vi "VI Properties Editor.vi"() -> ()   [LabVIEW 2023, in "VI Properties Editor.lvlib"]
doc: "Displays a window to add and edit properties of VIs in a streamlined way."
uses:
  VI Properties Editor.lvlib
  CTLs/VI Properties Editor State Data.ctl
  CTLs/VI Data.ctl
  CTLs/VI Properties.ctl
  <vilib>/picture/picture.llb/imagedata.ctl
  CTLs/Control Properties.ctl
  CTLs/VI Properties Editor Front Panel Controls.ctl
  CTLs/Config.ctl
  <vilib>/Utility/miscctls.llb/LVSelectionTypeDef.ctl
  <vilib>/ErrorRing/Error Ring.xnode
  SubVIs/FaKI SM.lvlib
panel:
  in  "Same Title as VI?":bool caption="Same as VI name"
  in  "Window Title":string
  in  "Add Copyright":bool
  out "Inline?":bool
  out "Reentrant?":bool
  in  "Prompt?":bool
  in  "Set all VIs":bool
  in  "error in (no error)":errorcluster
  in  "Controls":string[][](table)
  in  "Indicators":string[][](table)
  in  "Help Tag":string
  in  "Help Path":string
  out "Path to VI":string
  in  "VI Description":string
  out "VI Conn Pane":picture
  in  "Listbox with VIs":i32(listbox)=-1 caption="Select a VI to View/Edit Properties:"
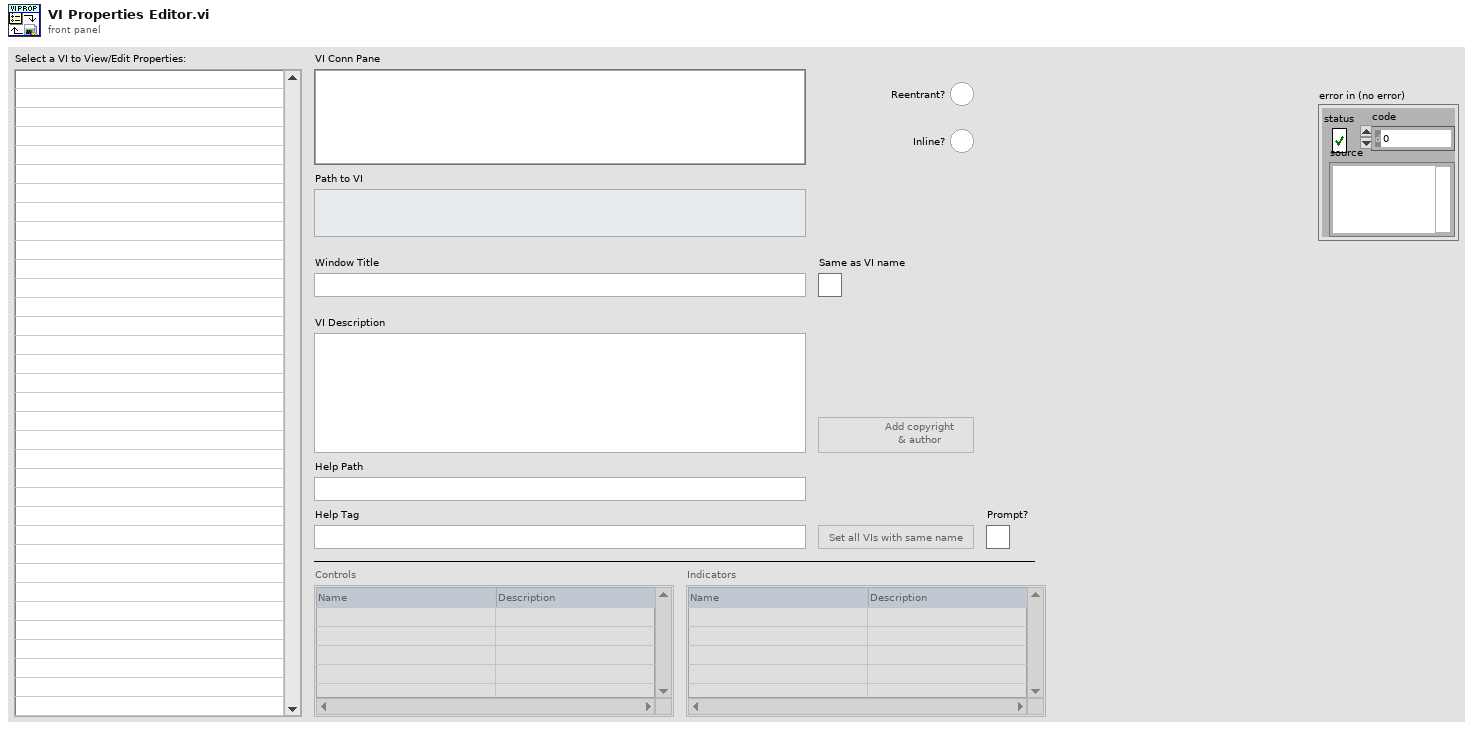
[diagram p1: front panel]
types:
  T1 = typedef "VI Properties Editor.lvlib/VI Properties Editor State Data.ctl" = cluster{"Core":cluster{"Current VI Reference":refnum<vi>, "Close Panel on Exit?":bool}, "New VI Data":T2[], "Saved VI Data":T2[], "Current Folder":path, "FP":T6, "Config Path":path, "Config":T7, "Desc Selection":T8}
  T2 = typedef "VI Properties Editor.lvlib/VI Data.ctl" = cluster{"VI":T3, "Ctl Properties":T5[]}
  T3 = typedef "VI Properties Editor.lvlib/VI Properties.ctl" = cluster{"Name":string, "Path":path, "Type":enum32{"invalid VI type", "Standard VI", "Control VI", "Global VI", "Polymorphic VI", "Configuration VI", "SubSystem", "Facade VI", "Method VI", "Statechart Diagram VI"}, "Window Title":string, "Description":string, "Help Path":path, "Help Tag":string, "Custom Title?":bool, "Reentrant?":bool, "Inlined?":bool, "Conpane Img":T4}
  T4 = typedef "imagedata.ctl" = cluster{"image type":i32, "image depth":i32, "image":u8[], "mask":u8[], "colors":u32[], "Rectangle":cluster{"left":i16, "top":i16, "right":i16, "bottom":i16}}
  T5 = typedef "VI Properties Editor.lvlib/Control Properties.ctl" = cluster{"UID":i32, "Name":string, "Description":string, "Tip Strip":string, "Is Indicator?":bool}
  T6 = typedef "VI Properties Editor.lvlib/VI Properties Editor Front Panel Controls.ctl" = cluster{"VI Selected":i32, "Help Path":string, "Help Tag":string, "VI Desc":string, "Controls":string[][], "Indicators":string[][], "Window Title":string, "Same Title?":bool}
  T7 = typedef "VI Properties Editor.lvlib/Config.ctl" = cluster{"Copyright Path":path, "Abbreviate Names?":bool, "Format Bold Text?":bool}
  T8 = typedef "LVSelectionTypeDef.ctl" = cluster{"Selection Start":u32, "Selection End":u32}
  T9 = enum32{"Invalid", "Standard", "Closed", "Hidden", "Minimized", "Maximized"}
  T10 = enum32{"invalid app kind", "Development System", "Run Time System", "Student Edition", "Embedded LabVIEW", "Evaluation", "Custom"}
  T11 = enum32{"invalid VI type", "Standard VI", "Control VI", "Global VI", "Polymorphic VI", "Configuration VI", "SubSystem", "Facade VI", "Method VI", "Statechart Diagram VI"}
  T12 = enum8{"Enabled", "Disabled", "Disabled and Grayed Out"}
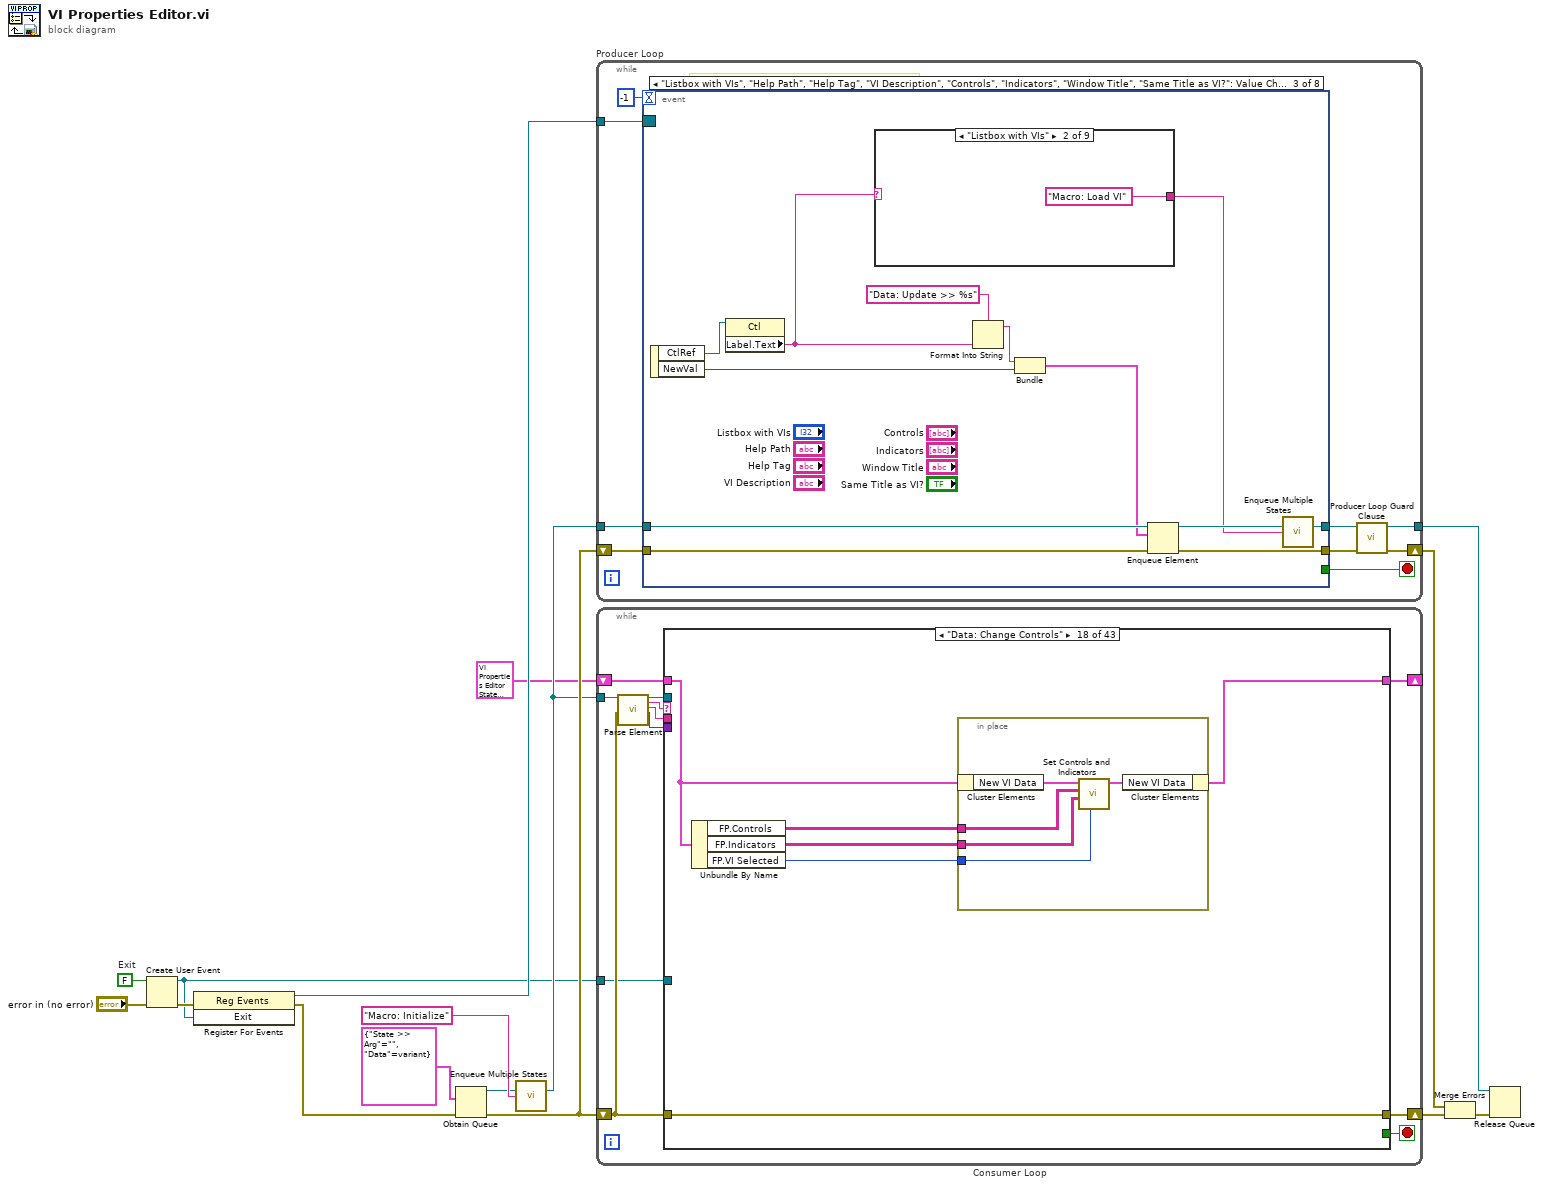
[diagram p0: block diagram]
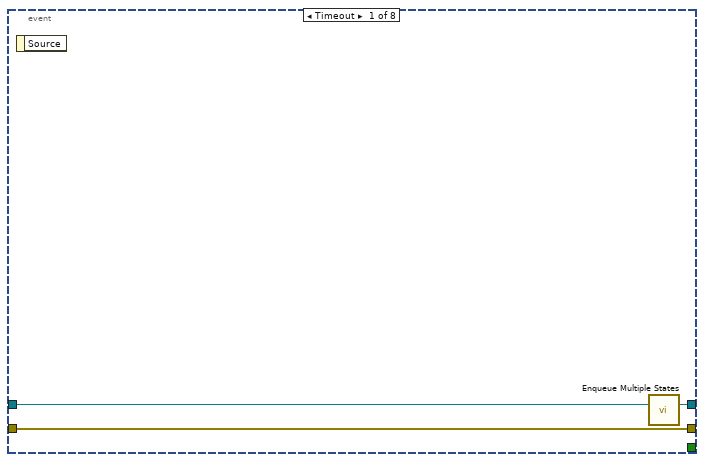
[diagram p2: hidden frame]
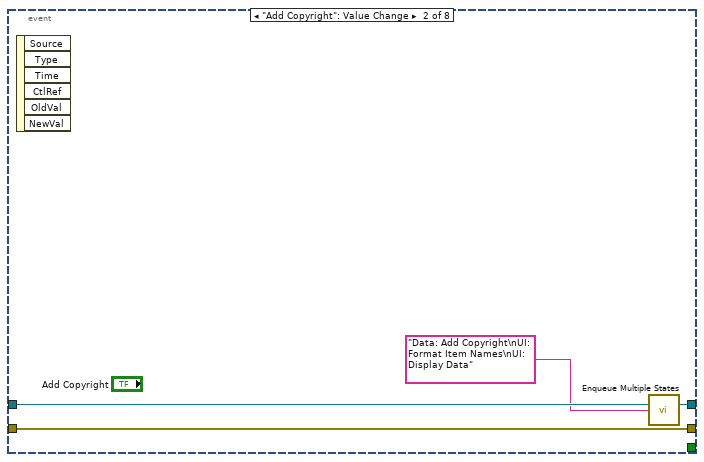
[diagram p3: hidden frame]
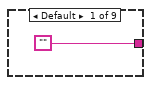
[diagram p4: hidden frame]
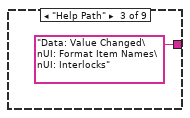
[diagram p5: hidden frame]
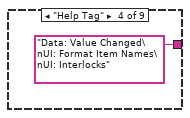
[diagram p6: hidden frame]
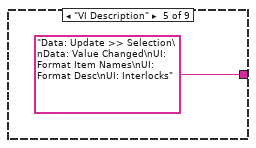
[diagram p7: hidden frame]
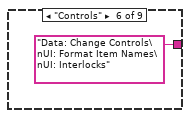
[diagram p8: hidden frame]
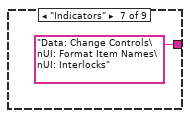
[diagram p9: hidden frame]
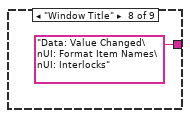
[diagram p10: hidden frame]
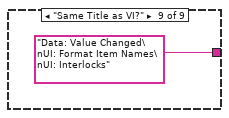
[diagram p11: hidden frame]
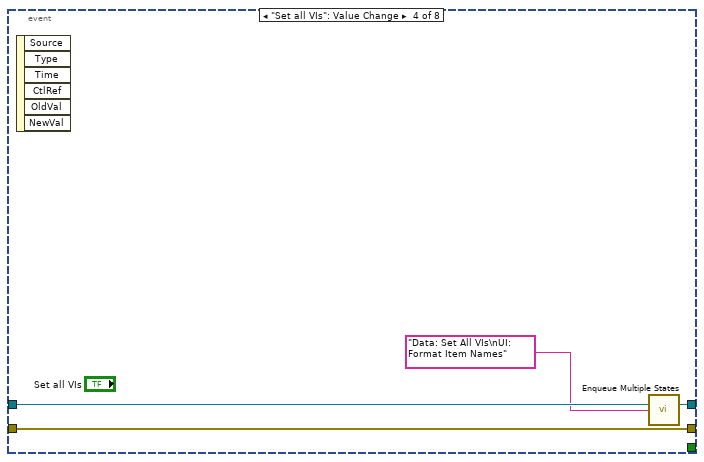
[diagram p12: hidden frame]
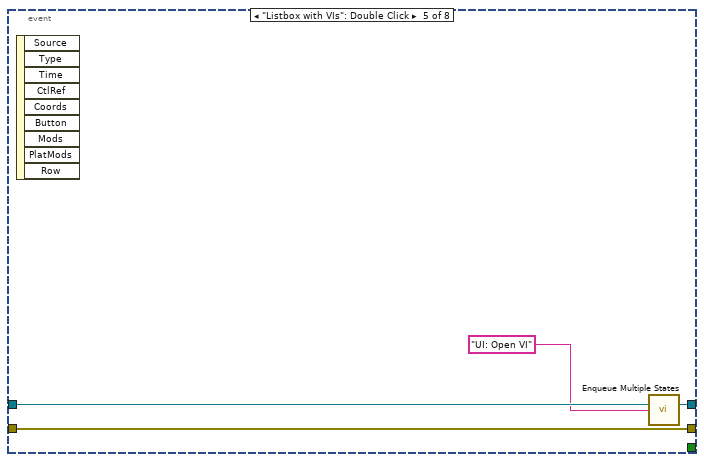
[diagram p13: hidden frame]
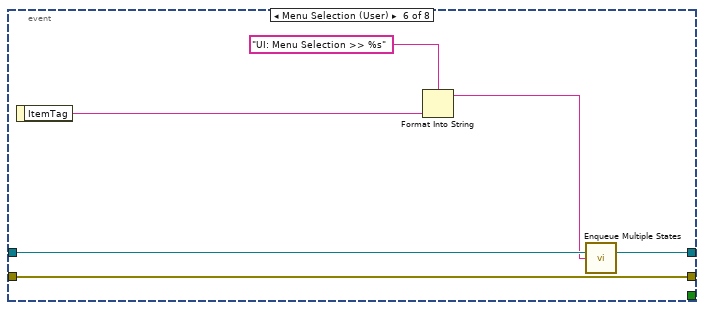
[diagram p14: hidden frame]
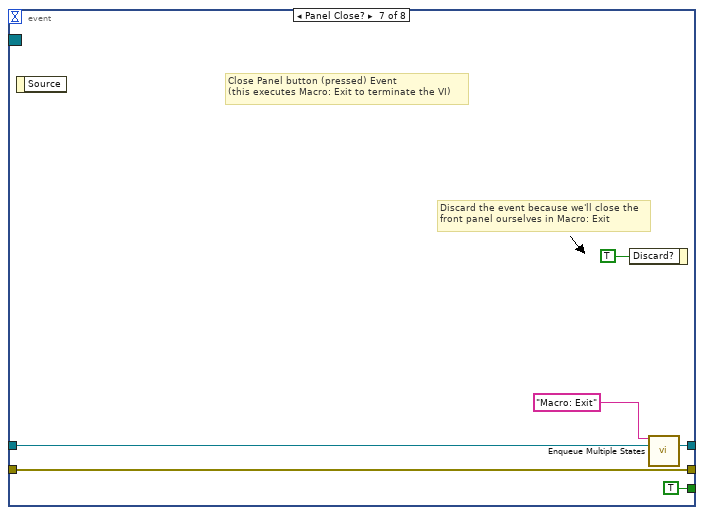
[diagram p15: hidden frame]
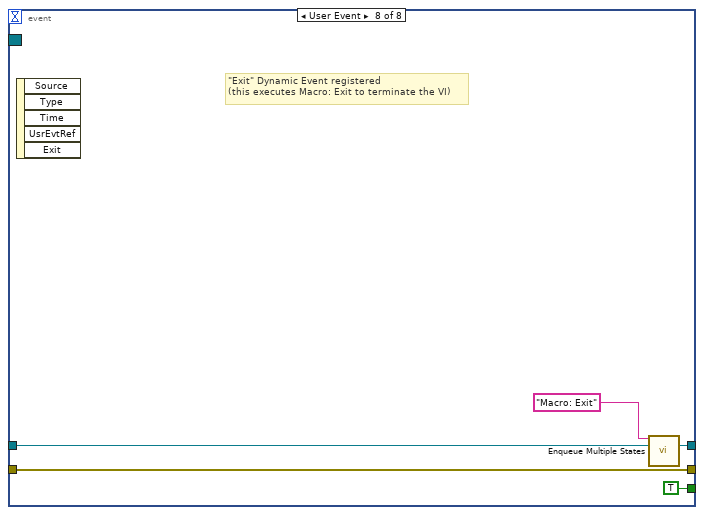
[diagram p16: hidden frame]
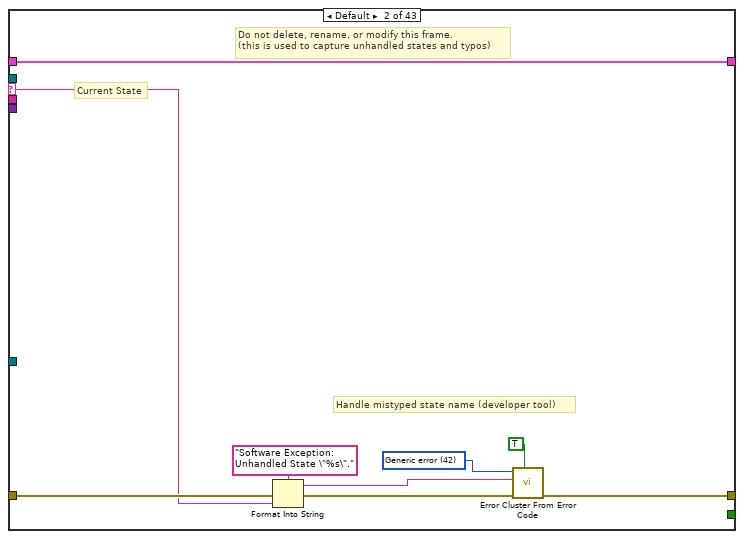
[diagram p18: hidden frame]
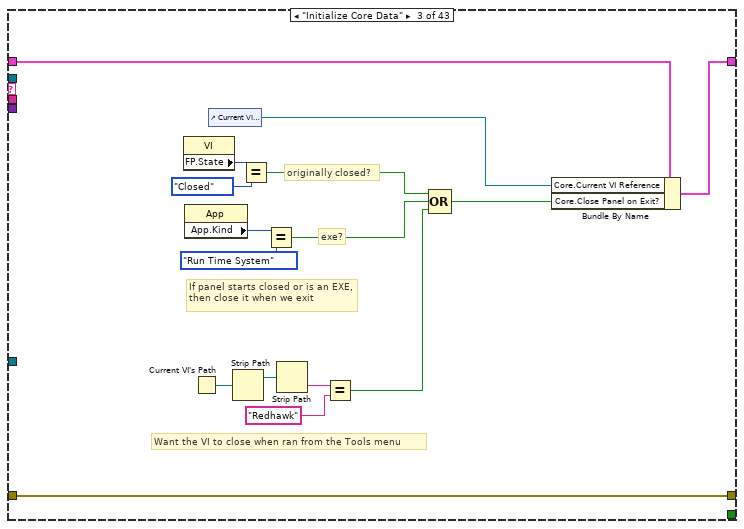
[diagram p19: hidden frame]
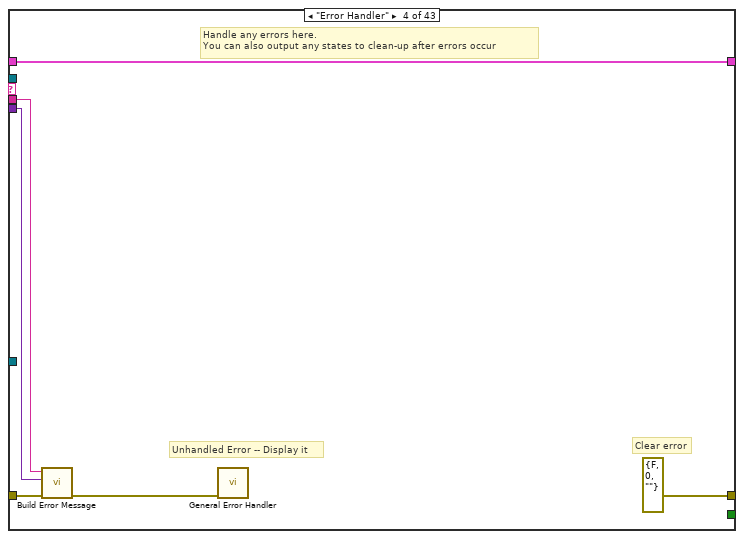
[diagram p20: hidden frame]
diagram:
  w6 = FALSE  # Exit
  n1 = Create User Event(user event datatype=w6, error in="error in (no error)") -> (user event=w3:refnum<user-event>, error out=w7:errorcluster)
  n2 = register-events(error in=w7, w3) -> (reference out=w4:refnum<event-registration>, error out=w5:errorcluster)  [unwired: 1 in]
  n3 = Obtain Queue(element data type=cluster{"State >> Arg":string, "Data":variant} {"State >> Arg"="", "Data"=variant}, error in (no error)=w5) -> (queue out=w13:refnum<queue>, error out=w16:errorcluster)  [unwired: 3 in, 1 out]
  n4 = call "Enqueue Multiple States.vi"("queue in"=w13, "State(s) at Back"="Macro: Initialize") -> ("queue out"=w12:refnum<queue>)  [unwired: 13 in]
  n5 = while "Producer Loop" {
    shift-right: [w20] -> w10
    shift-left: w16 -> [w25]
    tunnel: w4 -> [w17]
    tunnel: w12 -> [w23]
    tunnel: [w18] -> w8
    stop <- w22 stop-if-true
    # "executes when the state queue is empty"
    n6 = event shown="[2] \"Listbox with VIs\", \"Help Path\", \"Help Tag\", \"VI Description\", \"Controls\", \"Indicators\", \"Window Title\", \"Same Title as VI?\": Value Change" {
      selector: w17 -> [_ _ _ _ _ _ _ _]
      dyn-events: _ -> [_ _ _ _ _ _ _ _]
      timeout: -1 ("Timeout") -> [_ _ _ _ _ _ _ _]
      tunnel: [w26 w30 w42 w55 w59 w65 w73 w78] -> w21
      tunnel: w25 -> [w26 w30 w43 w55 w59 w65 w73 w78]
      tunnel: w23 -> [w27 w31 w41 w56 w60 w64 w70 w76]
      tunnel: [w28 w32 w44 w57 w61 w63 w69 w75] -> w19
      tunnel: [_ _ _ _ _ _ TRUE TRUE] -> w22
      event Timeout {
        n7 = event-data() -> ()  [unwired: 1 in, 1 out]
        n8 = call "Enqueue Multiple States.vi"("queue in"=w27) -> ("queue out"=w28:refnum<queue>)  [unwired: 14 in]
      }
      event "Add Copyright": Value Change {
        n9 = event-data() -> ()  [unwired: 1 in, 6 out]
        n10 = call "Enqueue Multiple States.vi"("queue in"=w31, "State(s) at Back"="Data: Add Copyright\nUI: Format Item Names\nUI: Display Data") -> ("queue out"=w32:refnum<queue>)  [unwired: 13 in]
      }
      event "Listbox with VIs", "Help Path", "Help Tag", "VI Description", "Controls", "Indicators", "Window Title", "Same Title as VI?": Value Change {
        n11 = event-data() -> ("CtlRef"=w39:refnum<vi>, "NewVal"=w33:variant)  [unwired: 1 in]
        n12 = property class="Ctl"(reference=w39) -> ("Label.Text"=w35:string)  [unwired: 1 in, 2 out]
        n13 = case shown="\"Listbox with VIs\"" w35 {
          tunnel: ["" "Macro: Load VI" "Data: Value Changed\nUI: Format Item Names\nUI: Interlocks" "Data: Value Changed\nUI: Format Item Names\nUI: Interlocks" "Data: Update >> Selection\nData: Value Changed\nUI: Format Item Names\nUI: Format Desc\nUI: Interlocks" "Data: Change Controls\nUI: Format Item Names\nUI: Interlocks" "Data: Change Controls\nUI: Format Item Names\nUI: Interlocks" "Data: Value Changed\nUI: Format Item Names\nUI: Interlocks" "Data: Value Changed\nUI: Format Item Names\nUI: Interlocks"] -> w34
          frame Default {
          }
          frame "Listbox with VIs" {
          }
          frame "Help Path" {
          }
          frame "Help Tag" {
          }
          frame "VI Description" {
          }
          frame "Controls" {
          }
          frame "Indicators" {
          }
          frame "Window Title" {
          }
          frame "Same Title as VI?" {
          }
        }
        n14 = Format Into String(format string="Data: Update >> %s", w35) -> (resulting string=w37:string)  [unwired: 2 in, 1 out]
        n15 = Bundle(w37, "NewVal"=w33) -> (w36:cluster{string, "NewVal":variant})  [unwired: 1 in]
        n16 = Enqueue Element(queue=w41, element=w36, error in (no error)=w43) -> (queue out=w40:refnum<queue>, error out=w42:errorcluster)  [unwired: 1 in, 1 out]
        n17 = call "Enqueue Multiple States.vi"("queue in"=w40, "State(s) at Back"=w34) -> ("queue out"=w44:refnum<queue>)  [unwired: 13 in]
      }
      event "Set all VIs": Value Change {
        n18 = event-data() -> ()  [unwired: 1 in, 6 out]
        n19 = call "Enqueue Multiple States.vi"("queue in"=w56, "State(s) at Back"="Data: Set All VIs\nUI: Format Item Names") -> ("queue out"=w57:refnum<queue>)  [unwired: 13 in]
      }
      event "Listbox with VIs": Double Click {
        n20 = event-data() -> ()  [unwired: 1 in, 9 out]
        n21 = call "Enqueue Multiple States.vi"("queue in"=w60, "State(s) at Back"="UI: Open VI") -> ("queue out"=w61:refnum<queue>)  [unwired: 13 in]
      }
      event Menu Selection (User) {
        n22 = event-data() -> ("ItemTag"=w66:string)  [unwired: 1 in]
        n23 = Format Into String(format string="UI: Menu Selection >> %s", w66) -> (resulting string=w62:string)  [unwired: 2 in, 1 out]
        n24 = call "Enqueue Multiple States.vi"("queue in"=w64, "State(s) at Back"=w62) -> ("queue out"=w63:refnum<queue>)  [unwired: 13 in]
      }
      event Panel Close? {
        # "Discard the event because we'll close the front panel ourselves in Macro: Exit"
        # "Close Panel button (pressed) Event\n(this executes Macro: Exit to terminate the VI)"
        n25 = event-data() -> ()  [unwired: 1 in, 1 out]
        n26 = event-data("Discard?"=TRUE) -> ()  [unwired: 1 in, 1 out]
        n27 = call "Enqueue Multiple States.vi"("State(s) at Front"="Macro: Exit", "queue in"=w70) -> ("queue out"=w69:refnum<queue>)  [unwired: 13 in]
      }
      event User Event {
        # "\"Exit\" Dynamic Event registered\n(this executes Macro: Exit to terminate the VI)"
        n28 = event-data() -> ()  [unwired: 1 in, 5 out]
        n29 = call "Enqueue Multiple States.vi"("State(s) at Front"="Macro: Exit", "queue in"=w76) -> ("queue out"=w75:refnum<queue>)  [unwired: 13 in]
      }
    }
    n30 = call "Producer Loop Guard Clause.vi"("error in (no error)"=w21, "queue in"=w19) -> ("error out"=w20:errorcluster, "queue out"=w18:refnum<queue>)  [unwired: 8 in]
  }
  n31 = while "Consumer Loop" {
    shift-right: [w86] -> _
    shift-left: T1 {"Core"={"Current VI Reference"=refnum, "Close Panel on Exit?"=FALSE}, "New VI Data"=[], "Saved VI Data"=[], "Current Folder"=path "", "FP"={"VI Selected"=0, "Help Path"="", "Help Tag"="", "VI Desc"="", "Controls"=[], "Indicators"=[], "Window Title"="", "Same Title?"=FALSE}, "Config Path"=path "", "Config"={"Copyright Path"=path "", "Abbreviate Names?"=FALSE, "Format Bold Text?"=FALSE}, "Desc Selection"={"Selection Start"=0, "Selection End"=0}} ("VI Properties Editor State Data") -> [w85]
    shift-right: [w89] -> w11
    shift-left: w16 -> [w88]
    tunnel: w12 -> [w84]
    tunnel: w3 -> [w79]
    stop <- w87 stop-if-true
    n32 = call "Parse Element.vi"("queue in"=w84, "error in (no error)"=w88) -> ("queue out"=w83:refnum<queue>, "State"=w82:string, "Arg"=w81:string, "Data"=w80:variant)  [unwired: 14 in]
    n33 = case shown="\"Data: Change Controls\"" w82 {
      selector: w82 -> [_ w92 _ _ _ _ _ _ _ _ _ _ _ _ _ _ _ _ _ _ _ _ _ _ _ _ _ _ _ _ _ _ _ _ _ _ _ _ _ _ _ _ _]
      tunnel: w83 -> [_ _ _ _ _ _ _ _ w268 _ _ _ _ _ _ _ _ _ _ _ _ _ _ w398 _ _ _ _ _ _ w595 _ _ _ _ _ _ _ w685 w689 w699 w709 w717]
      tunnel: w81 -> [_ _ _ w117 _ _ _ w146 _ _ _ _ _ _ _ _ _ _ w364 _ _ _ _ w393 w456 w464 w536 _ _ _ _ _ _ _ _ _ w647 _ _ _ w697 w707 _]
      tunnel: w85 -> [w90 w94 w111 w121 w124 w126 w137 w145 w264 w271 w278 w283 w292 w300 w306 w316 w338 w351 w367 w380 w384 w386 w389 w399 w457 w466 w541 w553 w561 w581 w591 w599 w608 w619 w630 w638 w645 w682 w686 w690 w700 w710 w721]
      tunnel: [w91 w99 w116 errorcluster {"status"=FALSE, "code"=0, "source"=""} ("error out") w125 w127 w130 w143 w266 w272 w280 w284 w293 w301 w304 w313 w339 w352 w373 w382 w385 w387 w391 w396 w458 w467 w537 w555 w556 w577 w584 w600 w609 w615 w626 w637 w650 w683 w687 w691 w701 w711 w722] -> w89
      tunnel: w88 -> [w91 w98 w116 w120 w125 w127 w129 w147 w267 w273 w275 w284 w293 w301 w305 w314 w339 w352 w369 w383 w385 w387 w392 w395 w459 w468 w538 w555 w556 w577 w593 w601 w610 w616 w627 w642 w649 w683 w687 w691 w701 w711 w722]
      tunnel: [_ _ _ _ TRUE _ _ _ _ _ _ _ _ _ _ _ _ _ _ _ _ _ _ _ _ _ _ _ _ _ _ _ _ _ _ _ _ _ _ _ _ _ _] -> w87
      tunnel: [w90 w94 w115 w121 w124 w126 w136 w142 w265 w271 w279 w282 w291 w299 w303 w317 w340 w353 w372 w380 w384 w386 w389 w399 w457 w466 w541 w553 w561 w581 w590 w599 w608 w618 w629 w638 w646 w682 w686 w690 w700 w710 w721] -> w86
      tunnel: w80 -> [_ _ _ w118 _ _ _ w144 _ _ _ _ _ _ _ _ _ _ _ _ _ _ _ _ _ _ _ _ _ _ _ _ _ _ _ _ _ _ _ _ _ _ _]
      tunnel: w79 -> [_ _ _ _ _ _ _ _ _ _ _ _ _ _ _ _ _ _ _ _ _ _ _ _ _ _ _ _ _ _ _ _ _ _ _ _ _ _ _ _ _ _ _]
      frame "---------- Core ----------" {
        # "Do not put any code in this frame.\n(it is a separator no-op)"
      }
      frame Default {
        w96 = 42 items=["No error", "Argument error", "Memory is full", "Out of zone", "End of file", "File already open", "Generic file I/O error", "File not found", "File permission error", "Disk is full", "Duplicate path", "Too many files open", "System feature not enabled", "Resource file not found", "Cannot add resource", "Resource not found", "Image not found", "Image memory error", "Pen does not exist", "Config type invalid", "Config token not found", "Config parse error", "Config memory error", "Bad external code format", "Bad external code offset", "External code not present", "Null window", "Destroy window error", "Null menu", "Print aborted", "Bad print record", "Print driver error", "Windows error during printing", "Memory error during printing", "Print dialog error", "Generic print error", "Invalid device refnum", "Device not found", "Device parameter error", "Device unit error", "Cannot open device", "Device call aborted", "Generic error", "Cancelled by user", "Object ID too low", "Object ID too high", "Object not in heap", "Unknown heap", "Unknown object (invalid DefProc)", "Unknown object (DefProc not in table)", "Message out of range", "Invalid (null) method", "Unknown message", "Manager call not supported", "Bad address", "Network operation in progress", "Network operation timed out", "Connection is busy", "Network attribute not supported", "Network error", "Address in use", "System out of memory", "Connection aborted", "Connection refused", "Not connected", "Already connected", "Connection closed", "Initialization error (interapplication manager)", "Bad occurrence", "Wait on unbound occurrence handler", "Occurrence queue overflow", "Datalog type conflict", "Unused", "Unrecognized type (interapplication manager)", "Memory corrupt", "Failed to make temporary DLL", "Old CIN version", "Drag socket not found", "Failed to load drop-object", "Failed to register OLE object", "Failed to release OLE object", "Format specifier type mismatch", "Unknown format specifier", "Too few format specifiers", "Too many format specifiers", "Scan failed", "Newer CIN version", "Error converting to variant", "Runtime menu error", "Password tampered", "Variant attribute not found", "Incompatible variant data type", "Event data is not available", "Event Store is not present", "Occurrence is not found", "Event Queue is not created", "Event info is not available", "Refnum passed is NULL", "Error retrieving Class GUID", "Error retrieving CoClass GUID", "Error retrieving TypeLib GUID.", "Bad built application magic bytes.", "Specific driver is different from the specific driver associated with the Logical Name.", "There is no session opened to the class driver.", "Max Error", "MAX - Error with config objects", "MAX - Error loading configuration", "MAX - Group not supported"]
        # "Current State"
        # "Do not delete, rename, or modify this frame.\n(this is used to capture unhandled states and typos)"
        # "Handle mistyped state name (developer tool)"
        n34 = Format Into String(format string="Software Exception: Unhandled State \"%s\"." ("message"), error in=w98, w92) -> (resulting string=w95:string, error out=w100:errorcluster)  [unwired: 1 in]
        n35 = call <vilib>:"Error Cluster From Error Code.vi"("show call chain? (False)"=TRUE, "error in (no error)"=w100, "error message (\"\")"=w95, "error code (0)"=w96) -> ("error out"=w99:errorcluster)  [unwired: 5 in]
      }
      frame "Initialize Core Data" {
        # "Want the VI to close when ran from the Tools menu"
        # "originally closed?"
        # "exe?"
        # "If panel starts closed or is an EXE, then close it when we exit"
        n36 = property class="VI"() -> ("FP.State"=w108:T9)  [unwired: 2 in, 2 out]
        n37 = property class="App"() -> ("App.Kind"=w114:T10)  [unwired: 2 in, 2 out]
        n38 = Current VI's Path() -> (path=w105:path)
        n39 = control-ref of="Current VI Reference"() -> (w109:refnum<vi>)
        n40 = Strip Path(path=w105) -> (stripped path=w104:path)  [unwired: 1 out]
        n41 = Equal?(x=w108, y=T9."Closed" ("Front Panel Window:State")) -> (x = y?=w106:bool)
        n42 = Equal?(x=w114, y=T10."Run Time System" ("Application:Kind")) -> (x = y?=w112:bool)
        n43 = Strip Path(path=w104) -> (name=w103:string)  [unwired: 1 out]
        n44 = Equal?(x=w103, y="Redhawk" ("name")) -> (x = y?=w101:bool)
        n45 = Compound Arithmetic op=OR(w106, w112, w101) -> (w110:bool)
        n46 = Bundle By Name(cluster=w111, "Core.Current VI Reference"=w109, "Core.Close Panel on Exit?"=w110) -> (w115:T1)
      }
      frame "Error Handler" {
        # "Unhandled Error -- Display it"
        # "Handle any errors here.\nYou can also output any states to clean-up after errors occur"
        # "Clear error"
        n47 = call "Build Error Message.vi"("error in (no error)"=w120, "Data"=w118, "Arg"=w117) -> ("error out"=w119:errorcluster)  [unwired: 8 in]
        n48 = call <vilib>:"General Error Handler.vi"("error in (no error)"=w119) -> ()  [unwired: 10 in, 5 out]
      }
      frame "Exit" {
        # "Do not put any code in this frame.\n(No errors that occur here will be handled.)"
      }
      frame "---------- Data ----------" {
        # "Do not put any code in this frame.\n(It is a separator no-op. You can make a copy of this frame to create a new Data frame)"
      }
      frame "Data: Initialize" {
        # "Initialize the shift-register data, here."
        n49 = call "Config Path--constant.vi"() -> ("Config Path"=w128:path)  [unwired: 11 in]
        n50 = Strip Path(path=w128) -> (stripped path=w134:path)  [unwired: 1 out]
        n51 = call <vilib>:"Check if File or Folder Exists.vi"("error in (no error)"=w129, "path"=w134) -> ("error out"=w133:errorcluster, "file or folder exists?"=w131:bool, "dup path"=w132:path)  [unwired: 7 in]
        n52 = case shown="False" w131 {
          tunnel: [w140 w141] -> w130
          tunnel: w133 -> [w139 w141]
          tunnel: w132 -> [w138 _]
          frame False {
            n53 = Create Folder(path (use dialog)=w138, error in=w139) -> (error out=w140:errorcluster)  [unwired: 1 in, 2 out]
          }
          frame True {
          }
        }
        n54 = Bundle By Name(cluster=w137, "FP.VI Selected"=-1, "Config Path"=w128) -> (w136:T1)
      }
      frame "Data: Update" {
        n55 = case shown="\"All Ctls\"" w146 {
          selector: w146 -> [w149 _ _ _ _ _ _ _ _ _ _ _ _ _]
          tunnel: w147 -> [_ w164 w167 w172 w178 w181 w194 w201 w208 w215 w227 w234 w241 w255]
          tunnel: w145 -> [w150 w161 w166 w171 w177 w180 w185 w198 w205 w212 w220 w232 w239 w256]
          tunnel: w144 -> [_ w163 _ _ _ _ w193 w200 w207 w214 w226 w233 w240 _]
          tunnel: [w148 w159 w167 w172 w178 w181 w190 w196 w203 w210 w224 w230 w237 w255] -> w143
          tunnel: [w150 w158 w165 w170 w175 w179 w189 w195 w202 w209 w223 w229 w236 w257] -> w142
          frame Default {
            n56 = xnode "Error Ring"("parameter 0"=w149) -> ("error out"=w148:errorcluster)
          }
          frame "Listbox with VIs" {
            n57 = Variant To Data(error in=w164, type=0, Variant=w163) -> (data=w160:i32, error out=w159:errorcluster)
            n58 = Bundle By Name(cluster=w161, "FP.VI Selected"=w160) -> (w158:T1)
          }
          frame "Abbr Names?" {
            n59 = in-place {
              n60 = in-place-cluster #1(w166) -> ("Config.Abbreviate Names?"=w169:bool)
              n61 = Not(x=w169) -> (.not. x?=w168:bool)
              n62 = in-place-cluster #1("Config.Abbreviate Names?"=w168) -> (w165:T1)
            }
          }
          frame "Format Bold?" {
            n63 = in-place {
              n64 = in-place-cluster #2(w171) -> ("Config.Format Bold Text?"=w174:bool)
              n65 = Not(x=w174) -> (.not. x?=w173:bool)
              n66 = in-place-cluster #2("Config.Format Bold Text?"=w173) -> (w170:T1)
            }
          }
          frame "Selection" {
            n67 = property on="VI Description" class="Str"() -> ("Text.Selection"=w176:T8)  [unwired: 2 in, 2 out]
            n68 = Bundle By Name(cluster=w177, "Desc Selection"=w176) -> (w175:T1)
          }
          frame "Inc Index" {
            n69 = in-place {
              n70 = in-place-cluster #3(w180) -> ("FP.VI Selected"=w183:i32)
              n71 = Increment(x=w183) -> (x+1=w182:i32)
              n72 = local write "Listbox with VIs"(w182) -> ()
              n73 = in-place-cluster #3("FP.VI Selected"=w182) -> (w179:T1)
            }
          }
          frame "Same Title as VI?" {
            n74 = Variant To Data(error in=w194, type=FALSE, Variant=w193) -> (data=w191:bool, error out=w190:errorcluster)
            n75 = Unbundle By Name(w185) -> ("New VI Data"=w188:T2[], "FP.VI Selected"=w187:i32)
            n76 = Index Array(array=w188, index=w187) -> (element=w186:T2)
            n77 = Unbundle By Name(w186) -> ("VI.Name"=w184:string)
            n78 = Bundle By Name(cluster=w185, "FP.Same Title?"=w191, "FP.Window Title"=w184) -> (w189:T1)
            n79 = local write "Window Title"(w184) -> ()
          }
          frame "Help Path" {
            n80 = Variant To Data(error in=w201, type="", Variant=w200) -> (data=w197:string, error out=w196:errorcluster)
            n81 = Bundle By Name(cluster=w198, "FP.Help Path"=w197) -> (w195:T1)
          }
          frame "Help Tag" {
            n82 = Variant To Data(error in=w208, type="", Variant=w207) -> (data=w204:string, error out=w203:errorcluster)
            n83 = Bundle By Name(cluster=w205, "FP.Help Tag"=w204) -> (w202:T1)
          }
          frame "VI Description" {
            n84 = Variant To Data(error in=w215, type="", Variant=w214) -> (data=w211:string, error out=w210:errorcluster)
            n85 = Bundle By Name(cluster=w212, "FP.VI Desc"=w211) -> (w209:T1)
          }
          frame "Window Title" {
            n86 = Unbundle By Name(w220) -> ("New VI Data"=w222:T2[], "FP.VI Selected"=w221:i32)
            n87 = Variant To Data(error in=w227, type="", Variant=w226) -> (data=w217:string, error out=w224:errorcluster)
            n88 = Index Array(array=w222, index=w221) -> (element=w219:T2)
            n89 = Unbundle By Name(w219) -> ("VI.Name"=w218:string)
            n90 = Equal?(x=w218, y=w217) -> (x = y?=w216:bool)
            n91 = Bundle By Name(cluster=w220, "FP.Window Title"=w217, "FP.Same Title?"=w216) -> (w223:T1)
            n92 = local write "Same Title as VI?"(w216) -> ()
          }
          frame "Controls" {
            n93 = Variant To Data(error in=w234, type=string[][] [], Variant=w233) -> (data=w231:string[][], error out=w230:errorcluster)
            n94 = Bundle By Name(cluster=w232, "FP.Controls"=w231) -> (w229:T1)
          }
          frame "Indicators" {
            n95 = Variant To Data(error in=w241, type=string[][] [], Variant=w240) -> (data=w238:string[][], error out=w237:errorcluster)
            n96 = Bundle By Name(cluster=w239, "FP.Indicators"=w238) -> (w236:T1)
          }
          frame "All Ctls" {
            n97 = Unbundle By Name(w256) -> ("New VI Data"=w254:T2[], "FP.VI Selected"=w253:i32)
            n98 = Index Array(array=w254, index=w253) -> (element=w252:T2)
            n99 = Unbundle By Name(w252) -> ("Ctl Properties"=w250:T5[], "VI.Help Tag"=w245:string, "VI.Help Path"=w247:path, "VI.Description"=w251:string, "VI.Window Title"=w244:string, "VI.Custom Title?"=w243:bool)
            n100 = call "Convert Controls to Arrays.vi"("Ctl Properties"=w250) -> ("Indicator Array"=w249:string[][], "Control Array"=w248:string[][])  [unwired: 9 in]
            n101 = Path To String(path=w247) -> (string=w246:string)
            n102 = Not(x=w243) -> (.not. x?=w242:bool)
            n103 = Bundle By Name(cluster=w256, "FP.Controls"=w248, "FP.Indicators"=w249, "FP.Help Tag"=w245, "FP.Help Path"=w246, "FP.VI Desc"=w251, "FP.Window Title"=w244, "FP.Same Title?"=w242) -> (w257:T1)
          }
        }
      }
      frame "Data: Read Config" {
        n104 = Unbundle By Name(w264) -> ("Config Path"=w263:path)
        n105 = call "Read Config.vi"("error in (no error)"=w267, "Path"=w263) -> ("error out"=w266:errorcluster, "Config"=w262:T7, "File Created?"=w261:bool)  [unwired: 7 in]
        n106 = Bundle By Name(cluster=w264, "Config"=w262) -> (w265:T1)
        n107 = Select(t="Data: Write Config", s=w261, f="") -> (s? t:f=w258:string)
        n108 = call "Enqueue Multiple States.vi"("queue in"=w268, "State(s) at Back"=w258) -> ()  [unwired: 13 in, 1 out]
      }
      frame "Data: Write Config" {
        n109 = Unbundle By Name(w271) -> ("Config Path"=w269:path, "Config"=w270:T7)
        n110 = call "Write Config.vi"("error in (no error)"=w273, "Config"=w270, "Path"=w269) -> ("error out"=w272:errorcluster)  [unwired: 8 in]
      }
      frame "Data: Load VIs" {
        n111 = Unbundle By Name(w278) -> ("Current Folder"=w274:path)
        n112 = property on="Listbox with VIs" class="LstBox (strict)"("Top Row"=0) -> ()  [unwired: 2 in, 2 out]
        n113 = call "Get All VI Data.vi"("error in (no error)"=w275, "Path"=w274) -> ("error out"=w280:errorcluster, "VI Data"=w277:T2[])  [unwired: 8 in]
        n114 = Bundle By Name(cluster=w278, "New VI Data"=w277, "Saved VI Data"=w277) -> (w279:T1)
      }
      frame "Data: Value Changed" {
        n115 = Unbundle By Name(w283) -> ("FP"=w281:T6)
        n116 = in-place {
          in-place-border: w281 -> [w286]
          n117 = in-place-cluster #4(w283) -> ("New VI Data"=w285:T2[])
          n118 = call "Set VI Properties.vi"("Front Panel Controls"=w286, "VI Data in"=w285) -> ("VI Data out"=w287:T2[])  [unwired: 9 in]
          n119 = in-place-cluster #4("New VI Data"=w287) -> (w282:T1)
        }
      }
      frame "Data: Revert Current" {
        n120 = Unbundle By Name(w292) -> ("FP.VI Selected"=w288:i32, "Saved VI Data"=w290:T2[])
        n121 = Index Array(array=w290, index=w288) -> (element=w289:T2)
        n122 = in-place {
          in-place-border: w289 -> [w296]
          in-place-border: w288 -> [w295]
          n123 = in-place-cluster #5(w292) -> ("New VI Data"=w297:T2[])
          n124 = Replace Array Subset(array=w297, new element=w296, index=w295) -> (w294:T2[])
          n125 = in-place-cluster #5("New VI Data"=w294) -> (w291:T1)
        }
      }
      frame "Data: Revert All" {
        n126 = Unbundle By Name(w300) -> ("Saved VI Data"=w298:T2[])
        n127 = in-place {
          in-place-border: w298 -> [w302]
          n128 = in-place-cluster #6(w300) -> ()  [unwired: 1 out]
          n129 = in-place-cluster #6("New VI Data"=w302) -> (w299:T1)
        }
      }
      frame "Data: Save All" {
        n130 = in-place {
          in-place-border: w305 -> [w312]
          in-place-border: [w311] -> w304
          n131 = in-place-cluster #7(w306) -> ("New VI Data"=w308:T2[], "Saved VI Data"=w307:T2[])
          n132 = call "Save All VI Data.vi"("error in (no error)"=w312, "Saved VI Data in"=w307, "New VI Data in"=w308) -> ("error out"=w311:errorcluster, "Saved VI Data out"=w309:T2[], "New VI Data out"=w310:T2[])  [unwired: 6 in]
          n133 = in-place-cluster #7("New VI Data"=w310, "Saved VI Data"=w309) -> (w303:T1)
        }
      }
      frame "Data: Save Current" {
        n134 = Unbundle By Name(w316) -> ("FP.VI Selected"=w315:i32)
        n135 = in-place {
          in-place-border: w315 -> [w322]
          in-place-border: w314 -> [w319]
          in-place-border: [w318] -> w313
          n136 = in-place-cluster #8(w316) -> ("New VI Data"=w324:T2[], "Saved VI Data"=w323:T2[])
          n137 = in-place {
            in-place-border: w319 -> [w326]
            in-place-border: [w325] -> w318
            n138 = in-place-array #9(w324, w322) -> (w334:T2)
            n139 = in-place-array #10(w323, w322) -> (w333:T2)
            n140 = Build Array(w334) -> (w332:T2[])
            n141 = Build Array(w333) -> (w331:T2[])
            n142 = call "Save All VI Data.vi"("error in (no error)"=w326, "Saved VI Data in"=w331, "New VI Data in"=w332) -> ("error out"=w325:errorcluster, "Saved VI Data out"=w328:T2[], "New VI Data out"=w330:T2[])  [unwired: 6 in]
            n143 = Index Array(array=w330) -> (element=w329:T2)  [unwired: 1 in]
            n144 = Index Array(array=w328) -> (element=w327:T2)  [unwired: 1 in]
            n145 = in-place-array #9(w329) -> (w320:T2[])  [unwired: 1 out]
            n146 = in-place-array #10(w327) -> (w321:T2[])  [unwired: 1 out]
          }
          n147 = in-place-cluster #8("New VI Data"=w320, "Saved VI Data"=w321) -> (w317:T1)
        }
      }
      frame "Data: Set All VIs" {
        n148 = Unbundle By Name(w338) -> ("FP.VI Selected"=w337:i32, "FP.VI Desc"=w335:string)
        n149 = in-place {
          in-place-border: w335 -> [w344]
          in-place-border: w337 -> [w345]
          in-place-border: "Prompt?" -> [w343]
          n150 = in-place-cluster #11(w338) -> ("New VI Data"=w346:T2[])
          n151 = Index Array(array=w346, index=w345) -> (element=w347:T2)
          n152 = Unbundle By Name(w347) -> ("VI.Path"=w342:path)
          n153 = call "Change All Descriptions.vi"("Prompt?"=w343, "New"=w344, "Path"=w342, "VI Data in"=w346) -> ("VI Data out"=w341:T2[])  [unwired: 5 in, 2 out]
          n154 = in-place-cluster #11("New VI Data"=w341) -> (w340:T1)
        }
      }
      frame "Data: Change Controls" {
        n155 = Unbundle By Name(w351) -> ("FP.Controls"=w350:string[][], "FP.Indicators"=w349:string[][], "FP.VI Selected"=w348:i32)
        n156 = in-place {
          in-place-border: w350 -> [w357]
          in-place-border: w349 -> [w356]
          in-place-border: w348 -> [w354]
          n157 = in-place-cluster #12(w351) -> ("New VI Data"=w358:T2[])
          n158 = call "Set Controls and Indicators.vi"("VI Index"=w354, "Indicators"=w356, "Controls"=w357, "VI Data In"=w358) -> ("VI Data Out"=w355:T2[])  [unwired: 7 in]
          n159 = in-place-cluster #12("New VI Data"=w355) -> (w353:T1)
        }
      }
      frame "Data: Add Copyright" {
        n160 = Unbundle By Name(w367) -> ("FP.VI Selected"=w361:i32, "Config.Copyright Path"=w366:path)
        n161 = Read from Text File(file (use dialog)=w366, error in=w369) -> (refnum out=w370:refnum<file>, text=w365:string, error out=w371:errorcluster)  [unwired: 2 in, 1 out]
        n162 = Equal?(x=w364, y="All") -> (x = y?=w362:bool)
        n163 = Close File(refnum=w370, error in=w371) -> (error out=w368:errorcluster)  [unwired: 1 out]
        n164 = Select(t=-1, s=w362, f=w361) -> (s? t:f=w359:i32)
        n165 = in-place {
          in-place-border: w368 -> [w378]
          in-place-border: [w377] -> w373
          in-place-border: w359 -> [w375]
          in-place-border: w365 -> [w374]
          n166 = in-place-cluster #13(w367) -> ("New VI Data"=w379:T2[])
          n167 = call "Add Copyright.vi"("error in (no error)"=w378, "Copyright Text"=w374, "VI Index"=w375, "VI Data"=w379) -> ("error out"=w377:errorcluster, "VI Data out"=w376:T2[])  [unwired: 6 in]
          n168 = in-place-cluster #13("New VI Data"=w376) -> (w372:T1)
        }
      }
      frame "Data: Cleanup" {
        # "Cleanup any data and references, here.\n(this is called automatically, by the Macro: Exit)"
        n169 = Unbundle By Name(w380) -> ("Core.Current VI Reference"=w381:refnum<vi>)
        n170 = Close Reference(reference=w381, error in (no error)=w383) -> (error out=w382:errorcluster)
      }
      frame "---------- UI ----------" {
        # "Do not put any code in this frame.\n(It is a separator no-op. You can make a copy of this frame to create a new UI frame)"
      }
      frame "UI: Initialize" {
        # "Initialize the User Interface, here.\n(this is called automatically, by the Macro: Init)"
      }
      frame "UI: Initialize Menu" {
        n171 = Unbundle By Name(w389) -> ("Config"=w388:T7)
        n172 = Current VI's Menubar() -> (w390:refnum<k9>)
        n173 = call "Initialize Menu Items.vi"("error in (no error)"=w392, "Config"=w388, "menu reference"=w390) -> ("error out"=w391:errorcluster)  [unwired: 8 in]
      }
      frame "UI: Menu Selection" {
        n174 = Current VI's Menubar() -> (w394:refnum<k9>)
        n175 = case shown="\"Format Bold Text\"" w393 {
          selector: w393 -> [w400 _ _ _ _ _ _ _ _ _ _ _ _ w440 w454]
          tunnel: ["" "UI: Select Folder" "UI: Edit Copyright" "Data: Revert Current\nUI: Format Item Names\nMacro: Load VI" "Data: Revert All\nUI: Format Item Names\nMacro: Load VI" "Data: Add Copyright >> All\nUI: Format Item Names\nUI: Display Data" "Macro: Save Current" "Macro: Save All" "UI: Focus Desc" "UI: Edit Copyright" "Macro: Save Current >> Go Next" "UI: Panel Updates >> Defer\nData: Update >> Selection\nUI: Format Desc >> Tags\nUI: Add Bold Tags\nData: Value Changed\nUI: Format Item Names\nUI: Format Desc\nUI: Panel Updates >> Undefer\nUI: Interlocks" "UI: Panel Updates >> Defer\nData: Update >> Selection\nUI: Format Desc >> Tags\nUI: Remove Bold Tags\nData: Value Changed\nUI: Format Item Names\nUI: Format Desc\nUI: Panel Updates >> Undefer\nUI: Interlocks" "Data: Update >> Abbr Names?\nUI: Format Item Names\nData: Write Config" w445] -> w397
          tunnel: w394 -> [_ _ _ _ _ _ _ _ _ _ _ _ _ w441 w455]
          tunnel: w395 -> [_ w410 w412 w414 w416 w418 w420 w422 w424 w426 w428 w430 w432 w435 w450]
          tunnel: [w401 w410 w412 w414 w416 w418 w420 w422 w424 w426 w428 w430 w432 w434 w449] -> w396
          frame Default {
            n176 = xnode "Error Ring"("parameter 0"=w400) -> ("error out"=w401:errorcluster)
          }
          frame "Open..." {
          }
          frame "Edit Copyright... " {
          }
          frame "Revert" {
          }
          frame "Revert All" {
          }
          frame "Add Copyright to All" {
          }
          frame "Save" {
          }
          frame "Save All" {
          }
          frame "Focus Desc Field" {
          }
          frame "Edit Copyright..." {
          }
          frame "Save and Edit Next Item" {
          }
          frame "Add Bold Tags" {
          }
          frame "Remove Bold Tags" {
          }
          frame "Abbr if Class in Lib" {
            n177 = Get Menu Item Info(7:w440, 8:w435, 11:w441) -> (0:w439:errorcluster, 3:w438:refnum<k9>, 4:w437:bool)  [unwired: 4 out]
            n178 = Not(x=w437) -> (.not. x?=w436:bool)
            n179 = Set Menu Item Info(6:w436, 7:w440, 8:w439, 11:w438) -> (0:w434:errorcluster)  [unwired: 3 in, 1 out]
          }
          frame "Format Bold Text" {
            n180 = Get Menu Item Info(7:w454, 8:w450, 11:w455) -> (0:w453:errorcluster, 3:w452:refnum<k9>, 4:w451:bool)  [unwired: 4 out]
            n181 = Not(x=w451) -> (.not. x?=w448:bool)
            n182 = Set Menu Item Info(6:w448, 7:w454, 8:w453, 11:w452) -> (0:w449:errorcluster)  [unwired: 3 in, 1 out]
            n183 = Select(t="UI: Format Desc", s=w448, f="UI: Format Desc >> Tags") -> (s? t:f=w443:string)
            n184 = Format Into String(format string="Data: Update >> Format Bold?\nData: Write Config\nUI: Display Data\n%s", w443) -> (resulting string=w445:string)  [unwired: 2 in, 1 out]
          }
        }
        n185 = call "Enqueue Multiple States.vi"("queue in"=w398, "State(s) at Back"=w397) -> ()  [unwired: 13 in, 1 out]
      }
      frame "UI: Cursor Set" {
        # "Argument"
        # "Set and Unset Cursor Busy.\n(Usage: \"UI: Cursor Set >> Busy|Idle\")"
        n186 = case shown="\"Idle\", Default" w456 {
          tunnel: w459 -> [w461 w463]
          tunnel: [w460 w462] -> w458
          frame "Idle", Default {
            n187 = call <vilib>:"Unset Busy.vi"("error in (no error)"=w461) -> ("error out"=w460:errorcluster)  [unwired: 10 in]
          }
          frame "Busy" {
            n188 = call <vilib>:"Set Busy.vi"("error in (no error)"=w463) -> ("error out"=w462:errorcluster)  [unwired: 9 in, 1 out]
          }
        }
      }
      frame "UI: Front Panel State" {
        # "Argument"
        # "Set Front Panel Open or Closed\n(Usage: \"UI: Front Panel State >> Open|Close\")"
        n189 = Unbundle By Name(w466) -> ("Core.Current VI Reference"=w465:refnum<vi>)
        n190 = case shown="\"Open\", \"Standard\", Default" w464 {
          tunnel: w468 -> [w475 w489 w501 w514 w527]
          tunnel: [w476 w490 w502 w515 w528] -> w467
          tunnel: w465 -> [w473 w487 w499 w512 w525]
          frame "Open", "Standard", Default {
            w469 = T9."Standard" ("State")
            n191 = property class="VI"(reference=w473, error in=w475) -> (reference out=w472:refnum<vi>, error out=w474:errorcluster, "FP.State"=w471:T9)
            n192 = Not Equal?(x=w471, y=w469) -> (x != y?=w470:bool)
            n193 = case shown="True" w470 {
              tunnel: [w481 w482] -> w476
              tunnel: w474 -> [w480 w482]
              tunnel: w472 -> [w478 _]
              tunnel: w469 -> [w477 _]
              frame True {
                n194 = invoke class="VI" method="FP.Open"(reference=w478, error in=w480, "Activate"=TRUE, "State"=w477) -> (error out=w481:errorcluster)  [unwired: 1 in, 4 out]
              }
              frame False {
              }
            }
          }
          frame "Close", "Closed" {
            n195 = property class="VI"(reference=w487, error in=w489) -> (reference out=w486:refnum<vi>, error out=w488:errorcluster, "FP.State"=w484:T9)
            n196 = Not Equal?(x=w484, y=T9."Closed" ("Front Panel Window:State")) -> (x != y?=w483:bool)
            n197 = case shown="True" w483 {
              tunnel: [w491 w494] -> w490
              tunnel: w488 -> [w491 w493]
              tunnel: w486 -> [_ w492]
              frame False {
              }
              frame True {
                n198 = invoke class="VI" method="FP.Close"(reference=w492, error in=w493) -> (error out=w494:errorcluster)  [unwired: 1 in, 2 out]
              }
            }
          }
          frame "Hidden", "Hide" {
            w495 = T9."Hidden" ("State")
            n199 = property class="VI"(reference=w499, error in=w501) -> (reference out=w498:refnum<vi>, error out=w500:errorcluster, "FP.State"=w497:T9)
            n200 = Not Equal?(x=w497, y=w495) -> (x != y?=w496:bool)
            n201 = case shown="True" w496 {
              tunnel: [w506 w507] -> w502
              tunnel: w500 -> [w505 w507]
              tunnel: w498 -> [w504 _]
              tunnel: w495 -> [w503 _]
              frame True {
                n202 = invoke class="VI" method="FP.Open"(reference=w504, error in=w505, "State"=w503) -> (error out=w506:errorcluster)  [unwired: 2 in, 4 out]
              }
              frame False {
              }
            }
          }
          frame "Minimize", "Minimized" {
            w508 = T9."Minimized" ("State")
            n203 = property class="VI"(reference=w512, error in=w514) -> (reference out=w511:refnum<vi>, error out=w513:errorcluster, "FP.State"=w510:T9)
            n204 = Not Equal?(x=w510, y=w508) -> (x != y?=w509:bool)
            n205 = case shown="True" w509 {
              tunnel: [w519 w520] -> w515
              tunnel: w513 -> [w518 w520]
              tunnel: w511 -> [w517 _]
              tunnel: w508 -> [w516 _]
              frame True {
                n206 = invoke class="VI" method="FP.Open"(reference=w517, error in=w518, "State"=w516) -> (error out=w519:errorcluster)  [unwired: 2 in, 4 out]
              }
              frame False {
              }
            }
          }
          frame "Maximize", "Maximized" {
            w521 = T9."Maximized" ("State")
            n207 = property class="VI"(reference=w525, error in=w527) -> (reference out=w524:refnum<vi>, error out=w526:errorcluster, "FP.State"=w523:T9)
            n208 = Not Equal?(x=w523, y=w521) -> (x != y?=w522:bool)
            n209 = case shown="True" w522 {
              tunnel: [w532 w533] -> w528
              tunnel: w526 -> [w531 w533]
              tunnel: w524 -> [w530 _]
              tunnel: w521 -> [w529 _]
              frame True {
                n210 = invoke class="VI" method="FP.Open"(reference=w530, error in=w531, "State"=w529) -> (error out=w532:errorcluster)  [unwired: 2 in, 4 out]
              }
              frame False {
              }
            }
          }
        }
      }
      frame "UI: Panel Updates" {
        n211 = Unbundle By Name(w541) -> ("Core.Current VI Reference"=w540:refnum<vi>)
        n212 = Equal?(x=w536, y="Defer") -> (x = y?=w534:bool)
        n213 = property class="VI"(reference=w540, error in=w538) -> (error out=w542:errorcluster, "Panel"=w539:refnum<vi>)  [unwired: 1 out]
        n214 = property class="Pnl"(reference=w539, error in=w542, "Defer Panel Updates"=w534) -> (error out=w537:errorcluster)  [unwired: 1 out]
      }
      frame "UI: Interlocks" {
        n215 = Unbundle By Name(w553) -> ("FP.VI Selected"=w544:i32, "New VI Data"=w545:T2[], "FP.VI Selected"=w554:i32)
        n216 = Current VI's Menubar() -> (w543:refnum<k9>)
        n217 = Index Array(array=w545, index=w554) -> (element=w552:T2)
        n218 = Greater Or Equal To 0?(x=w544) -> (x >= 0?=w547:bool)
        n219 = Unbundle By Name(w552) -> ("VI.Type"=w551:T11)
        n220 = call "UI Interlocks.vi"("menu reference"=w543, "VI Selected"=w544, "New VI Data"=w545) -> ()  [unwired: 8 in, 1 out]
        n221 = Equal?(x=w551, y=T11."Standard VI" ("x")) -> (x = y?=w549:bool)
        n222 = call "Gray if False.vi"("Grayed Out?"=w547) -> ("Enabled State"=w546:T12)  [unwired: 10 in]
        n223 = call "Gray if False.vi"("Grayed Out?"=w549) -> ("Enabled State"=w548:T12)  [unwired: 10 in]
        n224 = property on="Set all VIs" class="Bool"("DisabledEnum"=w546) -> ()  [unwired: 2 in, 2 out]
        n225 = property on="Add Copyright" class="Bool"("DisabledEnum"=w546) -> ()  [unwired: 2 in, 2 out]
        n226 = property on="Controls" class="Tbl (strict)"("DisabledEnum"=w548) -> ()  [unwired: 2 in, 2 out]
        n227 = property on="Indicators" class="Tbl (strict)"("DisabledEnum"=w548) -> ()  [unwired: 2 in, 2 out]
      }
      frame "UI: Format Item Names" {
        n228 = Unbundle By Name(w561) -> ("Config.Abbreviate Names?"=w557:bool, "New VI Data"=w560:T2[], "Saved VI Data"=w559:T2[])
        n229 = call "Format Item Names.vi"("Abbreviate Names?"=w557, "Saved VI Data"=w559, "New VI Data"=w560) -> ("Item Names"=w558:string[])  [unwired: 8 in]
        n230 = property on="Listbox with VIs" class="LstBox (strict)"("Item Names"=w558) -> ()  [unwired: 2 in, 2 out]
      }
      frame "UI: Display Data" {
        n231 = Unbundle By Name(w581) -> ("New VI Data"=w580:T2[], "FP.VI Selected"=w579:i32)
        n232 = Index Array(array=w580, index=w579) -> (element=w578:T2)
        n233 = Unbundle By Name(w578) -> ("Ctl Properties"=w576:T5[], "VI.Window Title"=w567:string, "VI.Description"=w572:string, "VI.Help Path"=w571:path, "VI.Help Tag"=w569:string, "VI.Custom Title?"=w566:bool, "VI.Path"=w564:path, "VI.Reentrant?"=→"Reentrant?":bool, "VI.Inlined?"=→"Inline?":bool, "VI.Conpane Img"=w568:T4)
        n234 = Path To String(path=w571) -> (string=w570:string)
        n235 = Not(x=w566) -> (.not. x?=w565:bool)
        n236 = call "Convert Controls to Arrays.vi"("Ctl Properties"=w576) -> ("Indicator Array"=w574:string[][], "Control Array"=w575:string[][])  [unwired: 9 in]
        n237 = Path To String(path=w564) -> (string=→"Path to VI":string)
        n238 = call <vilib>:"Draw Flattened Pixmap.vi"("image data"=w568) -> ("new picture"=→"VI Conn Pane":picture)  [unwired: 8 in]
        n239 = local write "Controls"(w575) -> ()
        n240 = local write "Indicators"(w574) -> ()
        n241 = local write "Window Title"(w567) -> ()
        n242 = local write "VI Description"(w572) -> ()
        n243 = local write "Help Path"(w570) -> ()
        n244 = local write "Help Tag"(w569) -> ()
        n245 = local write "Same Title as VI?"(w565) -> ()
      }
      frame "UI: Select Folder" {
        # "catch cancel error"
        n246 = call "File Dialog"("prompt"="Navigate to the directory of VIs to update:", "error in"=w593) -> ("selected path"=w589:path, "cancelled"=w588:bool, "error out"=w592:errorcluster)  [unwired: 10 in, 1 out]
        n247 = Select(t="", s=w588, f="UI: Cursor Set >> Busy\nData: Load VIs\nUI: Format Item Names\nUI: Cursor Set >> Idle") -> (s? t:f=w585:string)
        n248 = call "Enqueue Multiple States.vi"("queue in"=w595, "State(s) at Back"=w585) -> ()  [unwired: 13 in, 1 out]
        n249 = Bundle By Name(cluster=w591, "Current Folder"=w589) -> (w590:T1)
        n250 = call <vilib>:"Clear Errors.vi"("error in (no error)"=w592, "specific error code to clear (0: all)"=43) -> ("error out"=w584:errorcluster)  [unwired: 4 in, 1 out]
      }
      frame "UI: Open VI" {
        # "Open VI on DoubleClick"
        n251 = Unbundle By Name(w599) -> ("New VI Data"=w598:T2[], "FP.VI Selected"=w597:i32)
        n252 = Index Array(array=w598, index=w597) -> (element=w606:T2)
        n253 = Unbundle By Name(w606) -> ("VI.Path"=w596:path)
        n254 = Open VI Reference(vi path=w596, error in (no error)=w601) -> (vi reference=w603:refnum<vi>, error out=w602:errorcluster)  [unwired: 4 in]
        n255 = invoke class="VI" method="FP.Open"(reference=w603, error in=w602) -> (reference out=w605:refnum<vi>, error out=w604:errorcluster)  [unwired: 3 in, 3 out]
        n256 = Close Reference(reference=w605, error in (no error)=w604) -> (error out=w600:errorcluster)
      }
      frame "UI: Edit Copyright" {
        n257 = Unbundle By Name(w608) -> ("Config.Copyright Path"=w607:path)
        n258 = Format Into String(format string="Notepad.exe %s", error in=w610, w607) -> (resulting string=w613:string, error out=w614:errorcluster)  [unwired: 1 in]
        n259 = call <vilib>:"System Exec.vi"("wait until completion? (T)"=FALSE, "error in (no error)"=w614, "command line"=w613) -> ("error out"=w609:errorcluster)  [unwired: 5 in, 3 out]
      }
      frame "UI: Add Bold Tags" {
        n260 = control-ref of="VI Description"() -> (w624:refnum<vi>)
        n261 = property class="Str"(reference=w624, error in=w616) -> (reference out=w621:refnum<vi>, error out=w625:errorcluster, "Value"=w623:string, "Text.Selection"=w622:T8)
        n262 = call "Add Bold Tags.vi"("Selection in"=w622, "Value in"=w623) -> ("Selection out"=w620:T8, "Value out"=w617:string)  [unwired: 8 in]
        n263 = property class="Str"(reference=w621, error in=w625, "Value"=w617, "Text.Selection"=w620) -> (error out=w615:errorcluster)  [unwired: 1 out]
        n264 = Bundle By Name(cluster=w619, "FP.VI Desc"=w617) -> (w618:T1)
      }
      frame "UI: Remove Bold Tags" {
        n265 = control-ref of="VI Description"() -> (w635:refnum<vi>)
        n266 = property class="Str"(reference=w635, error in=w627) -> (reference out=w632:refnum<vi>, error out=w636:errorcluster, "Value"=w634:string, "Text.Selection"=w633:T8)
        n267 = call "Remove Bold Tags.vi"("Selection in"=w633, "Value in"=w634) -> ("Selection out"=w631:T8, "Value out"=w628:string)  [unwired: 8 in]
        n268 = property class="Str"(reference=w632, error in=w636, "Value"=w628, "Text.Selection"=w631) -> (error out=w626:errorcluster)  [unwired: 1 out]
        n269 = Bundle By Name(cluster=w630, "FP.VI Desc"=w628) -> (w629:T1)
      }
      frame "UI: Focus Desc" {
        n270 = control-ref of="VI Description"() -> (w641:refnum<vi>)
        n271 = property class="Str"(reference=w641, error in=w642, "Key Focus"=TRUE, "Text.Selection Start"=u32 4294967295 ("Text.Selection:End")) -> (error out=w637:errorcluster)  [unwired: 1 out]
      }
      frame "UI: Format Desc" {
        n272 = control-ref of="VI Description"() -> (w648:refnum<vi>)
        n273 = Unbundle By Name(w645) -> ("Config.Format Bold Text?"=w644:bool, "Desc Selection"=w643:T8)
        n274 = in-place {
          in-place-border: [w658] -> w650
          in-place-border: w649 -> [w657]
          in-place-border: w648 -> [w656]
          in-place-border: w647 -> [w655]
          in-place-border: w644 -> [w652]
          in-place-border: w643 -> [w651]
          n275 = in-place-cluster #14(w645) -> ("FP.VI Desc"=w654:string)
          n276 = case shown="\"Style\", Default" w655 {
            tunnel: [w659 w675] -> w658
            tunnel: w657 -> [w662 w674]
            tunnel: w656 -> [w661 w673]
            tunnel: w654 -> [_ w671]
            tunnel: [w668 w671] -> w653
            tunnel: w652 -> [w667 w672]
            tunnel: w651 -> [_ w670]
            frame "Tags" {
              n277 = call "Reset Plain Formatting.vi"("error in (no error)"=w662, "Str Refnum"=w661) -> ("error out"=w663:errorcluster, "Str Refnum out"=w660:refnum<vi>)  [unwired: 8 in]
              n278 = call "Find Bold Formatting.vi"("error in (no error)"=w663, "Str Refnum"=w660) -> ("error out"=w669:errorcluster, "Length"=w664:i32[], "Start"=w665:i32[], "Str Refnum out"=w666:refnum<vi>)  [unwired: 6 in]
              n279 = call "Replace Formatting with Tags.vi"("Set Value? (T)"=w667, "error in (no error)"=w669, "Length"=w664, "Start"=w665, "Str Refnum"=w666) -> ("error out"=w659:errorcluster, "New String"=w668:string)  [unwired: 4 in, 1 out]
            }
            frame "Style", Default {
              n280 = case shown="True" w672 {
                tunnel: [w676 w681] -> w675
                tunnel: w674 -> [w676 w680]
                tunnel: w673 -> [_ w679]
                tunnel: w671 -> [_ w678]
                tunnel: w670 -> [_ w677]
                frame False {
                }
                frame True {
                  n281 = call "Bold Description String.vi"("error in (no error)"=w680, "Text.Selection"=w677, "String"=w678, "Str Refnum"=w679) -> ("error out"=w681:errorcluster)  [unwired: 7 in]
                }
              }
            }
          }
          n282 = in-place-cluster #14("FP.VI Desc"=w653) -> (w646:T1)
        }
      }
      frame "---------- Macro ----------" {
        # "Do not put any code in this frame.\n(It is a separator no-op. You can make a copy of this frame to create a new Macro frame)"
      }
      frame "Macro: Initialize" {
        w684 = "Data: Initialize\nInitialize Core Data\nData: Read Config\nUI: Initialize\nUI: Interlocks\nUI: Front Panel State >> Open\nUI: Initialize Menu"  # Data: Initialize Initialize Core Data Data: Read Config UI: Initialize UI: Interlocks UI: Front Panel State >> Open UI: Initialize Menu
        # "Initialization Macro\n(This is called once, when the VI starts)"
        n283 = call "Enqueue Multiple States.vi"("State(s) at Front"=w684, "queue in"=w685) -> ()  [unwired: 13 in, 1 out]
      }
      frame "Macro: Load VI" {
        n284 = call "Enqueue Multiple States.vi"("State(s) at Front"="UI: Panel Updates >> Defer\nData: Update >> All Ctls\nUI: Display Data\nUI: Format Desc\nUI: Panel Updates >> Undefer\nUI: Interlocks\nUI: Focus Desc", "queue in"=w689) -> ()  [unwired: 13 in, 1 out]
      }
      frame "Macro: Save All" {
        n285 = Equal?(x=w697, y="Close") -> (x = y?=w695:bool)
        n286 = Select(t="Macro: Exit", s=w695, f="") -> (s? t:f=w692:string)
        n287 = call "Enqueue Multiple States.vi"("State(s) at Front"="UI: Cursor Set >> Busy\nData: Save All\nUI: Format Item Names\nUI: Interlocks\nUI: Cursor Set >> Idle", "queue in"=w699, "State(s) at Back"=w692) -> ()  [unwired: 12 in, 1 out]
      }
      frame "Macro: Save Current" {
        n288 = Equal?(x=w707, y="Go Next") -> (x = y?=w705:bool)
        n289 = Select(t="Data: Update >> Inc Index\nMacro: Load VI", s=w705, f="") -> (s? t:f=w702:string)
        n290 = call "Enqueue Multiple States.vi"("State(s) at Front"="UI: Cursor Set >> Busy\nData: Save Current\nUI: Format Item Names\nUI: Interlocks\nUI: Cursor Set >> Idle", "queue in"=w709, "State(s) at Back"=w702) -> ()  [unwired: 12 in, 1 out]
      }
      frame "Macro: Exit" {
        # "Exit Macro\n(This is called once, when the VI exits)"
        n291 = Unbundle By Name(w721) -> ("Core.Close Panel on Exit?"=w720:bool)
        n292 = invoke class="VI" method="Default Vals.Reinit All"() -> ()  [unwired: 3 in, 3 out]
        n293 = property on="Listbox with VIs" class="LstBox (strict)"("Top Row"=0) -> ()  [unwired: 2 in, 2 out]
        n294 = property on="Listbox with VIs" class="LstBox (strict)"("Item Names"=string[] []) -> ()  [unwired: 2 in, 2 out]
        n295 = Select(t="UI: Front Panel State >> Close\n", s=w720, f="") -> (s? t:f=w716:string)
        n296 = Concatenate Strings(w716, "Data: Cleanup\nExit") -> (w714:string)
        n297 = call "Enqueue Multiple States.vi"("State(s) at Front"=w714, "queue in"=w717) -> ()  [unwired: 13 in, 1 out]
      }
    }
  }
  n298 = Merge Errors(w10, w11) -> (w9:errorcluster)
  n299 = Release Queue(queue=w8, error in (no error)=w9) -> ()  [unwired: 1 in, 3 out]
